vi "Make JSON Object.vi"(6 "Pretty Print?":bool, 8 "error in (no error)":errorcluster, 9 "JSON elements":string[](array[string]), 11 "Names":string[](array[string])) -> (0 "error out":errorcluster, 3 "JSON Object Text out":string)   [LabVIEW 2015, in "JSONtext.lvlib"]
doc: "Format a JSON Object from named JSON elements."
uses:
  JSONtext.lvlib
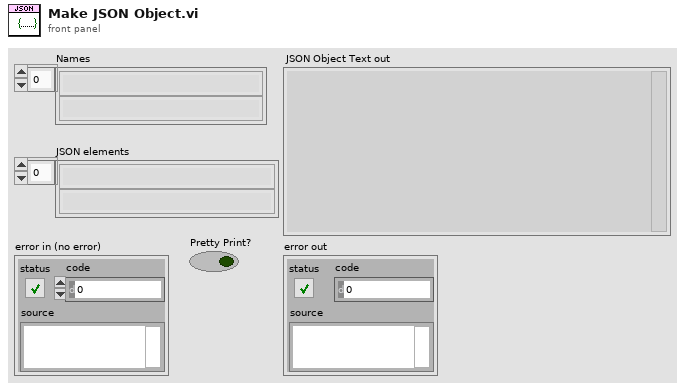
[diagram p1: front panel]
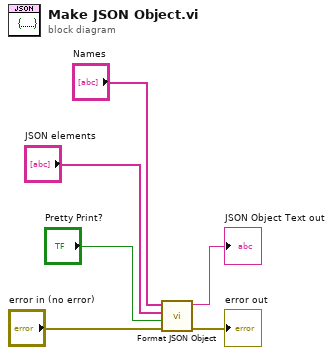
[diagram p0: block diagram]
diagram:
  n1 = call "Format JSON Object.vi"("error in (no error)"="error in (no error)", "Pretty Print?"="Pretty Print?", "JSON elements"="JSON elements", "Names"="Names") -> ("error out"=→"error out":errorcluster, "JSON Object Text out"=→"JSON Object Text out":string)  [unwired: 6 in]
